vi "XYs_to_Intensity.vi"(8 "error in (no error)":errorcluster, 11 "XYs in":cluster{"X-array":dbl[], "Y-array":dbl[]}[](array[cluster])) -> (0 "error out":errorcluster, 3 "Intensity data (y) out":dbl[][](array[numeric]))   [LabVIEW 2016]
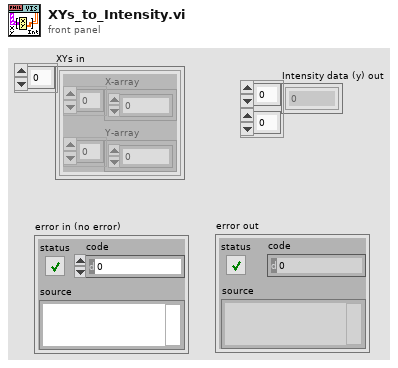
[diagram p1: front panel]
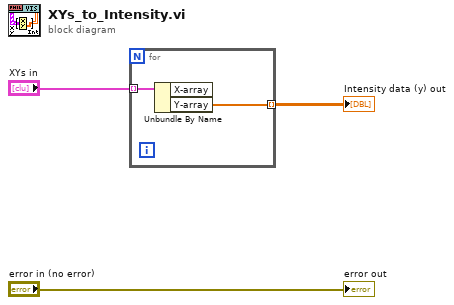
[diagram p0: block diagram]
diagram:
  n1 = for {
    tunnel: "XYs in" -> [w5] mode=indexing
    tunnel: [w4] -> w1 mode=indexing
    n2 = Unbundle By Name(w5) -> ("Y-array"=w4:dbl[])  [unwired: 1 out]
  }
  "Intensity data (y) out" <- w1
  "error out" <- "error in (no error)"
